vi "Get Setpoint Tag Path.vi"(11 "channel Name":string) -> (3 "tag path":string)   [LabVIEW 2020, in "FlexLoggerTagHelpers.lvlib"]
uses:
  FlexLoggerTagHelpers.lvlib
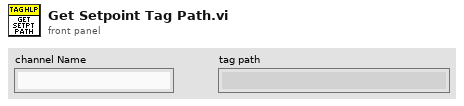
[diagram p1: front panel]
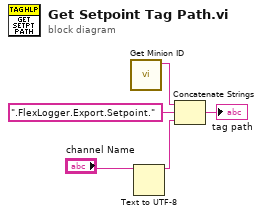
[diagram p0: block diagram]
diagram:
  n1 = call <vilib>:"Get Minion ID.vi"() -> ("minion id"=w4:string)  [unwired: 11 in]
  n2 = Text to UTF-8(11:"channel Name") -> (3:w1:string)  [unwired: 2 in, 1 out]
  n3 = Concatenate Strings(w4, ".FlexLogger.Export.Setpoint." ("string"), w1) -> (→"tag path":string)
